vi "toml_list_keys.vi"(4 "vi":refnum<vi>, 7 "section":string, 8 "error in (no error)":errorcluster, 11 "path in":path) -> (0 "error out":errorcluster, 1 "keys":string[](array[string]), 2 "section exists":bool, 3 "path out":path)   [LabVIEW 2017]
uses:
  <vilib>/Utility/error.llb/Clear Errors.vi
  toml_lock_obtain.vi
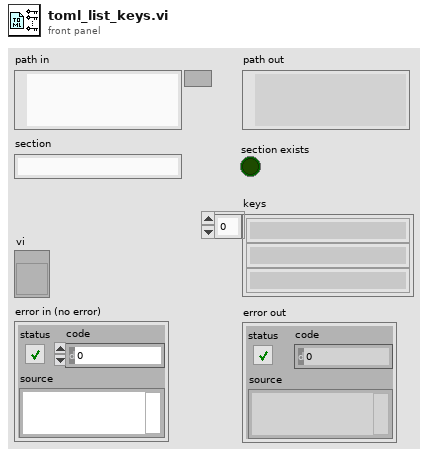
[diagram p1: front panel]
types:
  T1 = enum16{"open", "replace", "create", "open or create", "replace or create", "replace or create with confirmation"}
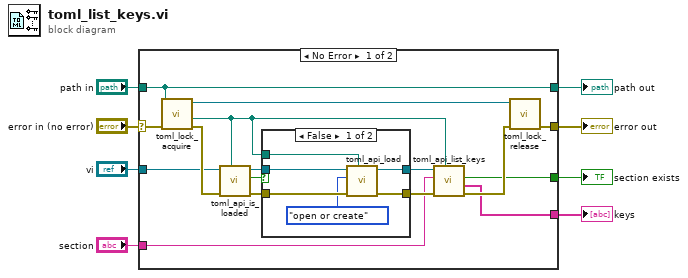
[diagram p0: block diagram]
diagram:
  n1 = case shown="No Error" "error in (no error)" {
    selector: "error in (no error)" -> [w23 w33]
    tunnel: [w22 w33] -> w7
    tunnel: "vi" -> [w11 _]
    tunnel: "path in" -> [w21 w34]
    tunnel: [w21 w34] -> w4
    tunnel: [w13 _] -> w3
    tunnel: [w12 _] -> w2
    tunnel: "section" -> [w9 _]
    frame No Error {
      n2 = call "toml_lock_acquire.vi"("error in (no error)"=w23, "path in"=w21) -> ("error out"=w17:errorcluster, "resolved path"=w10:path, "lock"=w24:refnum<queue>)  [unwired: 7 in]
      n3 = call "toml_api_is_loaded.vi"("resolved path"=w10, "error in (no error)"=w17, "vi in"=w11) -> ("error out"=w19:errorcluster, "file loaded"=w20:bool, "vi out"=w18:refnum<vi>)  [unwired: 5 in, 1 out]
      n4 = case shown="False" w20 {
        tunnel: w19 -> [w30 w32]
        tunnel: [w29 w32] -> w16
        tunnel: w10 -> [w26 _]
        tunnel: w18 -> [w28 w31]
        tunnel: [w27 w31] -> w15
        frame False {
          n5 = call "toml_api_load.vi"("resolved path"=w26, "error in (no error)"=w30, "operation"=T1."open or create" ("operation (open or create)"), "vi in"=w28) -> ("error out"=w29:errorcluster, "vi out"=w27:refnum<vi>)  [unwired: 5 in, 1 out]
        }
        frame True {
        }
      }
      n6 = call "toml_api_list_keys.vi"("resolved path"=w10, "error in (no error)"=w16, "section"=w9, "vi in"=w15) -> ("error out"=w14:errorcluster, "keys"=w12:string[], "section exists"=w13:bool)  [unwired: 4 in, 1 out]
      n7 = call "toml_lock_release.vi"("error in (no error)"=w14, "lock"=w24) -> ("error out"=w22:errorcluster)  [unwired: 9 in]
    }
    frame Error {
    }
  }
  "error out" <- w7
  "path out" <- w4
  "section exists" <- w3
  "keys" <- w2
